vi "GSP_Shutter_ControlGUI.vi"(4 "error in (no error)":errorcluster) -> (0 "error out":errorcluster)   [LabVIEW 2015]
uses:
  coll_actions.ctl
panel:
  in  "GO":bool
  in  "Exposure (ms)":i32=200
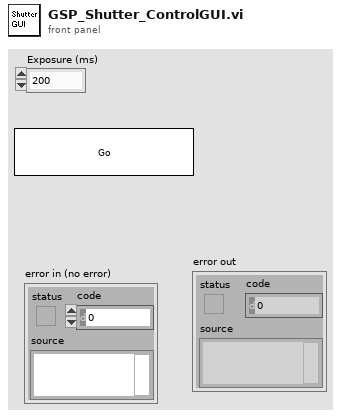
[diagram p1: front panel]
types:
  T1 = typedef "coll_actions.ctl" = enum16{"Launch", "Move", "Home", "Open Shutter", "Close Shutter", "Shutdown"}
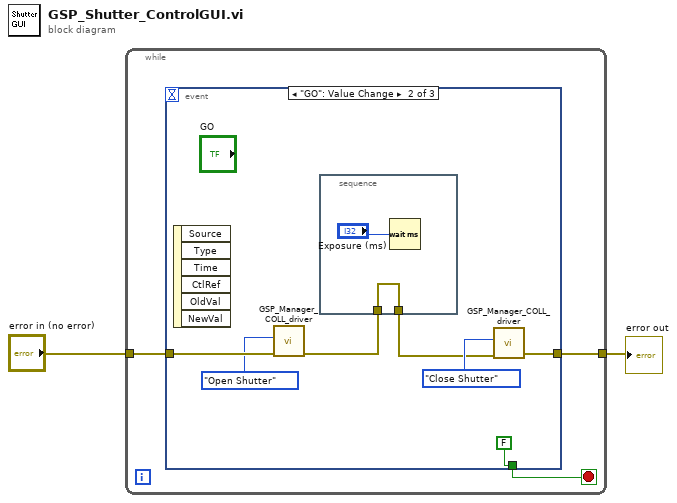
[diagram p0: block diagram]
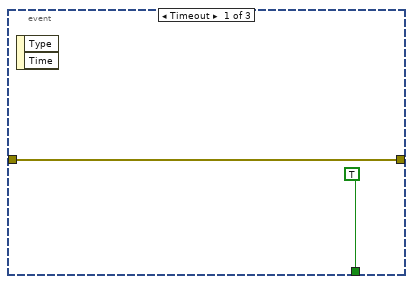
[diagram p2: hidden frame]
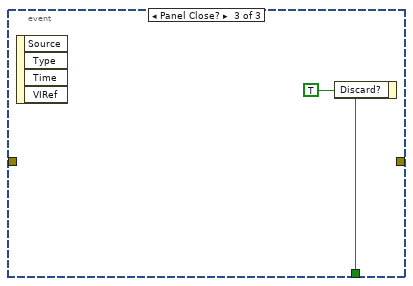
[diagram p3: hidden frame]
diagram:
  n1 = while {
    tunnel: "error in (no error)" -> [w5]
    tunnel: [w4] -> w1
    stop <- w3 stop-if-true
    n2 = event shown="[1] \"GO\": Value Change" {
      selector: _ -> [_ _ _]
      dyn-events: _ -> [_ _ _]
      timeout: _ -> [_ _ _]
      tunnel: w5 -> [w7 w13 _]
      tunnel: [w7 w10 _] -> w4
      tunnel: [TRUE FALSE w17] -> w3
      event Timeout {
        n3 = event-data() -> ()  [unwired: 1 in, 2 out]
      }
      event "GO": Value Change {
        n4 = event-data() -> ()  [unwired: 1 in, 6 out]
        n5 = call "GSP_Manager_COLL_driver.vi"("error in (no error)"=w13, "Action"=coll_actions."Open Shutter") -> ("error out"=w9:errorcluster)  [unwired: 4 in, 1 out]
        n6 = stacked-sequence {
          tunnel: w9 -> [w15]
          tunnel: [w15] -> w8
          frame #0 {
            n7 = Wait (ms)(milliseconds to wait="Exposure (ms)") -> ()  [unwired: 1 out]
          }
        }
        n8 = call "GSP_Manager_COLL_driver.vi"("error in (no error)"=w8, "Action"=coll_actions."Close Shutter") -> ("error out"=w10:errorcluster)  [unwired: 4 in, 1 out]
      }
      event Panel Close? {
        w17 = TRUE
        n9 = event-data() -> ()  [unwired: 1 in, 4 out]
        n10 = event-data("Discard?"=w17) -> ()  [unwired: 1 in, 1 out]
      }
    }
  }
  "error out" <- w1
